vi "Periodic Tasks.vi"(7 "Chassis X SPD":dbl=0.65, 8 "error in":errorcluster) -> ()   [LabVIEW 2019]
doc: "This VI runs in parallel to other tasks. It can contain as many user-defined periodic loops as you need. These can carry out PID or other sorts of timed response."
uses:
  Robot Global Data.vi
  <vilib>/Rock Robotics/Network Tables/NT Write Number.vi
  <vilib>/Analysis/NI_AALPro.lvlib
  <vilib>/Rock Robotics/Network Tables/NT Write Boolean.vi
  <vilib>/Rock Robotics/WPI/RobotDrive/WPI_RobotDriveArcadeDrive_Standard(NoSaturation).vi
  <vilib>/Rock Robotics/Network Tables/NT Read Number.vi
panel:
  in  "Chassis Y SPD":dbl=0.65
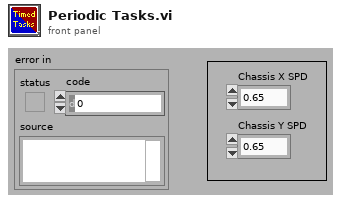
[diagram p1: front panel]
types:
  T1 = typedef "WPI_MotorControlDeviceRef.ctl" = cluster{"DeviceStatus":errorcluster, "Type":T2, "PWM":cluster{"PWM Channel":T3, "DeadBand":T4}, "CAN":cluster{"Device Number":u8, "SetOutput VI Ref":variant, "GetOutput VI Ref":variant, "Enable VI Ref":variant, "Disable VI Ref":variant, "Data":variant}, "Invert":bool, "DIO PWM":cluster{"PWM \"Enable\" Channel":T3, "DIOChannel":T5, "PWM Rate":dbl}}
  T2 = typedef "WPI_MotorControlType.ctl" = enum16{"PWM", "CAN", "DIO PWM"}
  T3 = typedef "FPGA_DIOPWMChannel.ctl" = enum8{"PWM 0", "PWM 1", "PWM 2", "PWM 3", "PWM 4", "PWM 5", "PWM 6", "PWM 7", "PWM 8", "PWM 9", "PWM MXP 0", "PWM MXP 1", "PWM MXP 2", "PWM MXP 3", "PWM MXP 4", "PWM MXP 5", "PWM MXP 6", "PWM MXP 7", "PWM MXP 8", "PWM MXP 9", "Invalid"}
  T4 = typedef "WPI_PWMDeadband.ctl" = cluster{"Name":string, "maxPositivePwm":i32, "minPositivePwm":i32, "centerPwm":i32, "maxNegativePwm":i32, "minNegativePwm":i32, "angularRange":u16}
  T5 = typedef "FPGA_DIOChannel.ctl" = enum8{"DIO 0", "DIO 1", "DIO 2", "DIO 3", "DIO 4", "DIO 5", "DIO 6", "DIO 7", "DIO 8", "DIO 9", "DIO MXP 0", "DIO MXP 1", "DIO MXP 2", "DIO MXP 3", "DIO MXP 4", "DIO MXP 5", "DIO MXP 6", "DIO MXP 7", "DIO MXP 8", "DIO MXP 9", "DIO MXP 10", "DIO MXP 11", "DIO MXP 12", "DIO MXP 13", "DIO MXP 14", "DIO MXP 15", "SPI Port CS1", "SPI Port CS2", "SPI Port CS3", "SPI Port MISO", "SPI Port MOSI", "Invalid"}
  T6 = typedef "WPI_JoystickDevRef.ctl" = cluster{"Device":T7}
  T7 = typedef "WPI_JoystickDeviceEnum.ctl" = enum16{"USB 0", "USB 1", "USB 2", "USB 3", "USB 4", "USB 5"}
  T8 = typedef "WPI_RobotDriveDevRef.ctl" = cluster{"DevStatus":errorcluster, "Motors[]":T1[], "Square Inputs":bool, "Max Output":dbl}
  T9 = cluster{"JoystickDevRef":T6, "RobotDriveDevRef":T8}
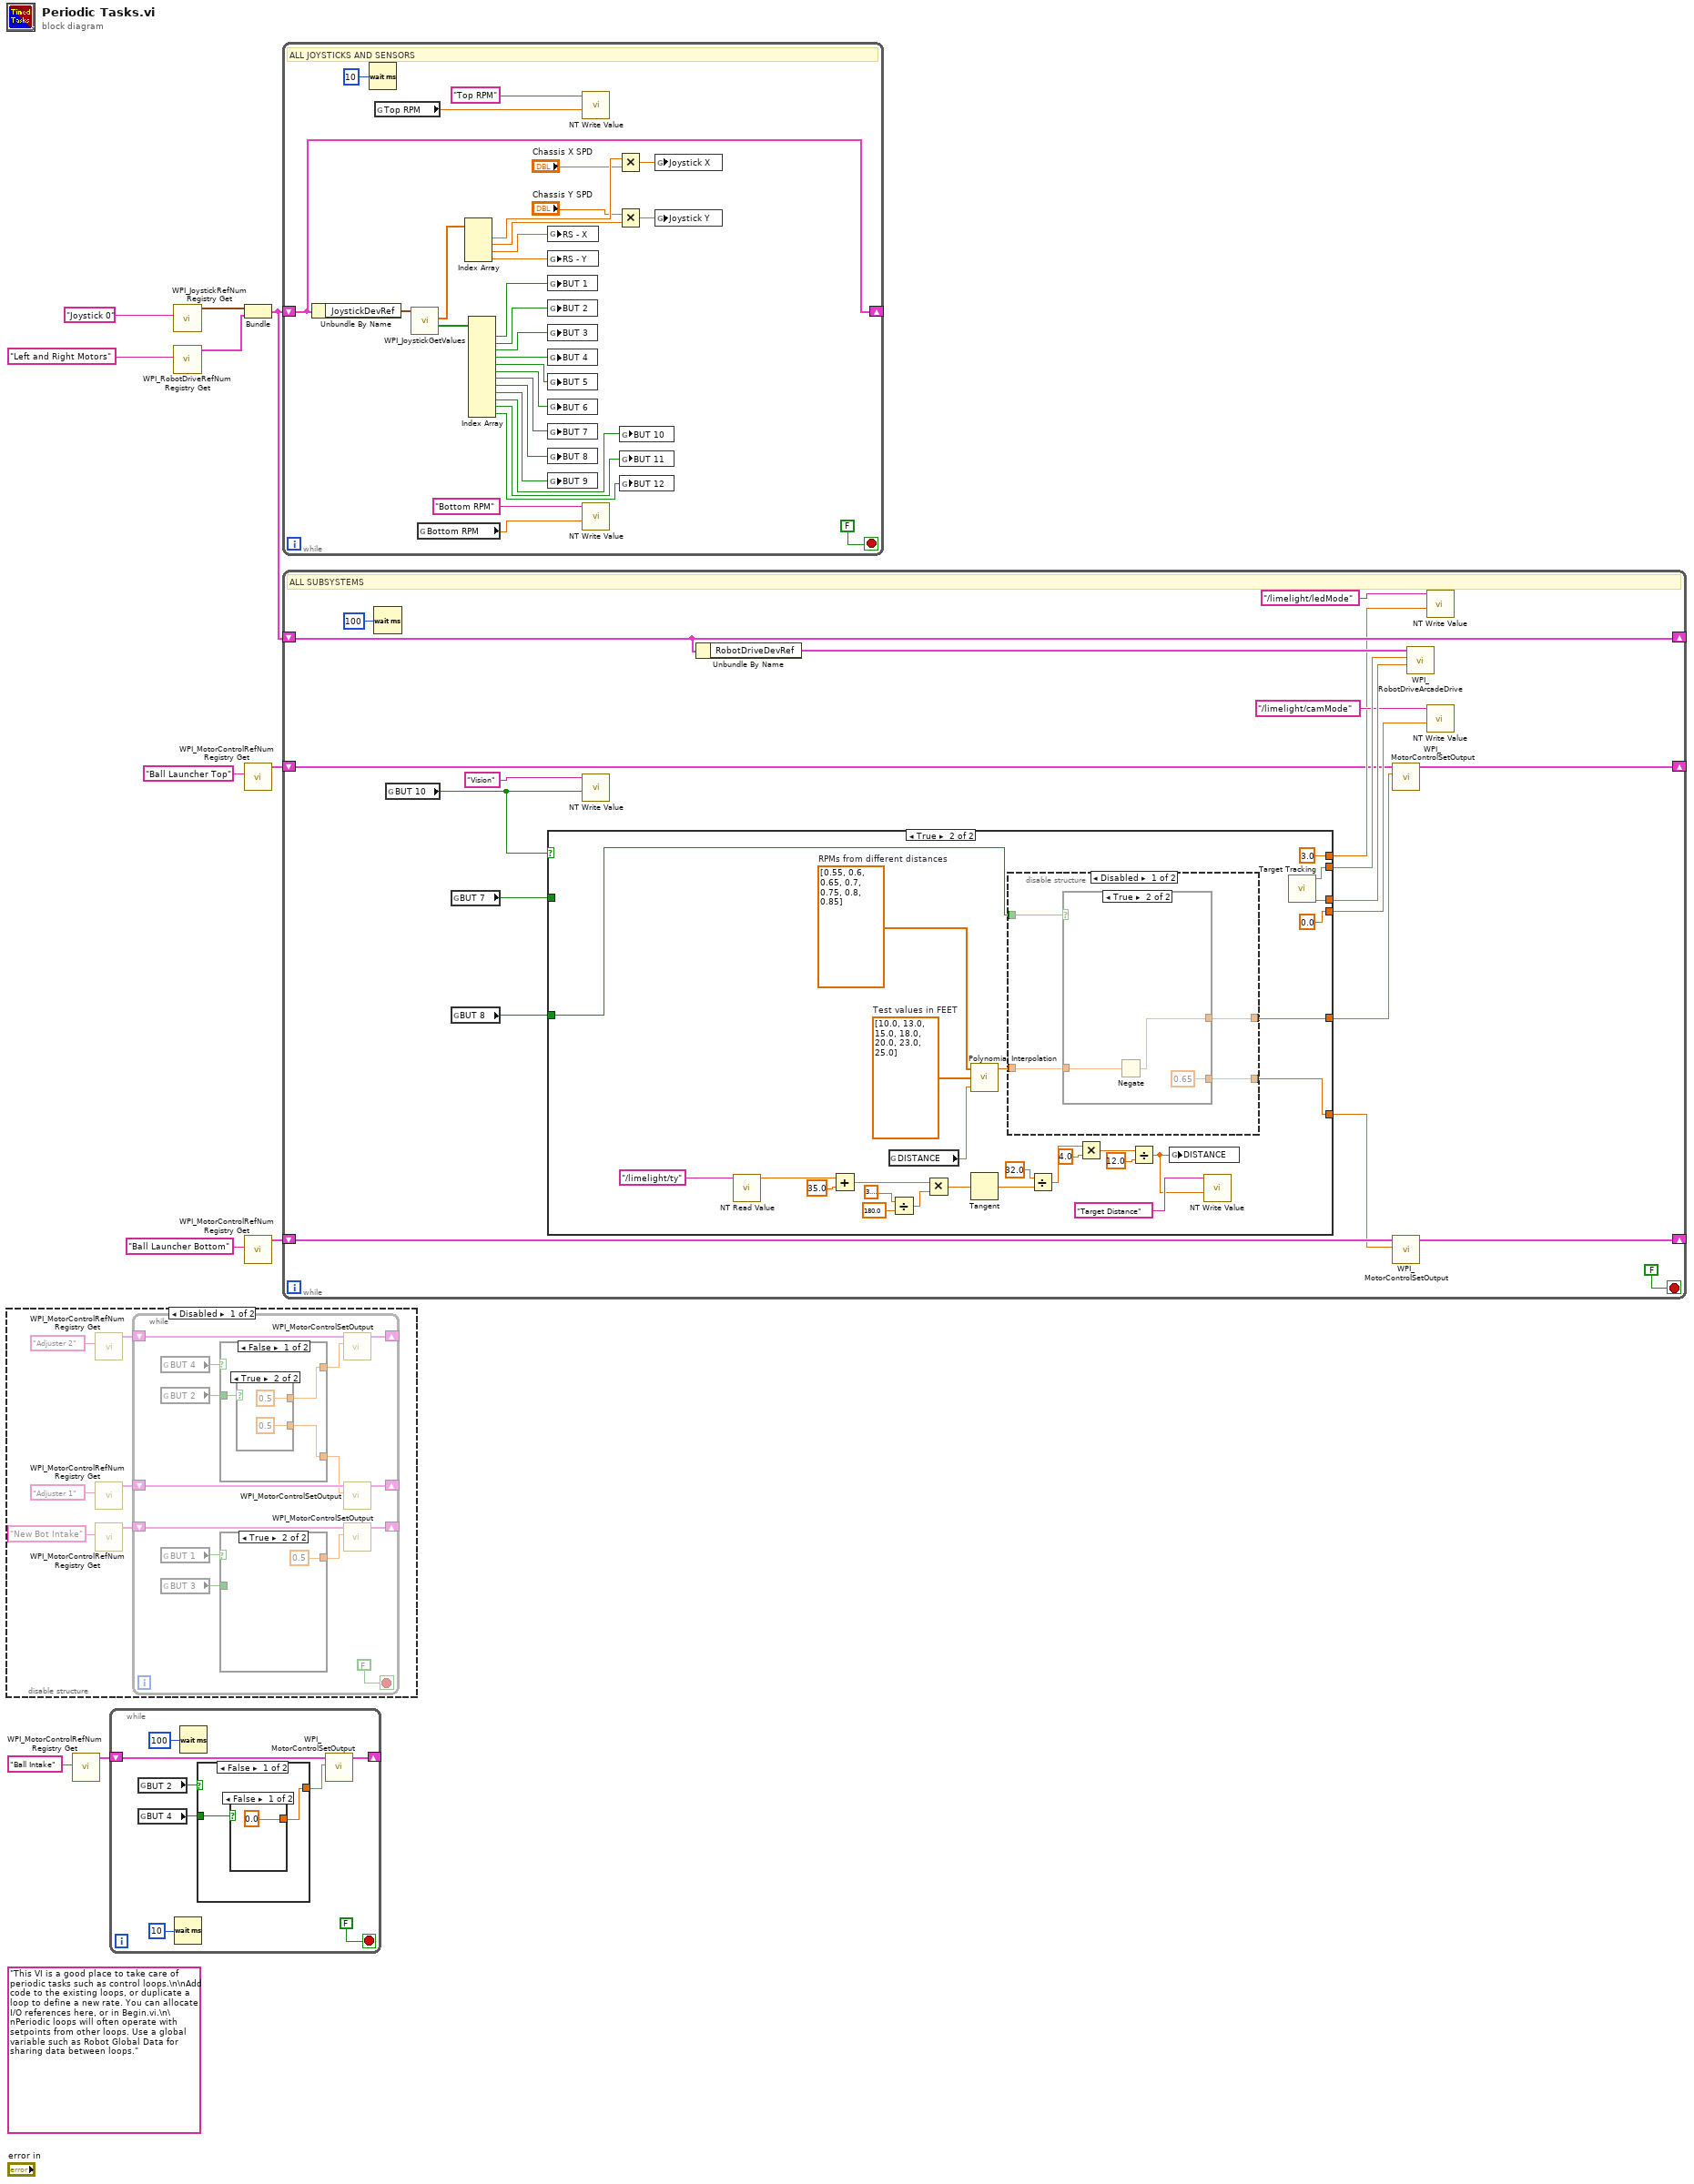
[diagram p0: block diagram]
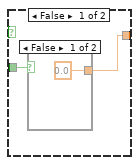
[diagram p2: hidden frame]
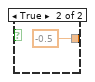
[diagram p3: hidden frame]
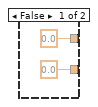
[diagram p4: hidden frame]
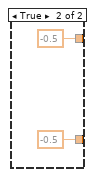
[diagram p5: hidden frame]
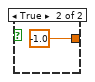
[diagram p7: hidden frame]
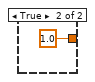
[diagram p8: hidden frame]
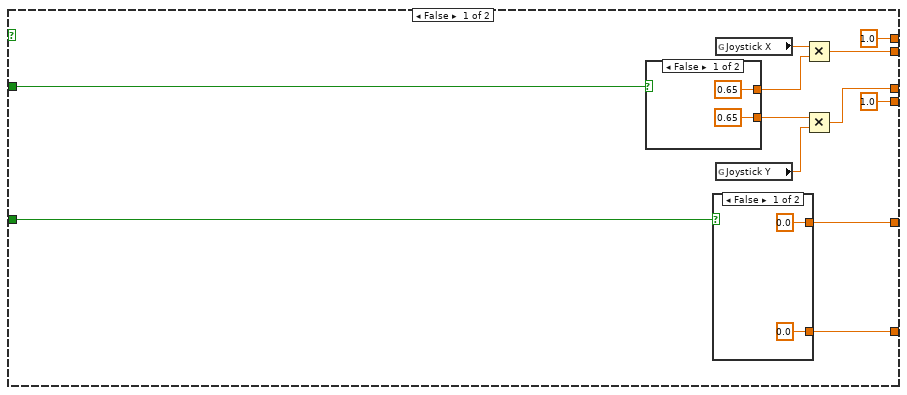
[diagram p9: hidden frame]
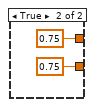
[diagram p10: hidden frame]
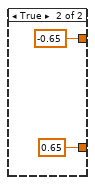
[diagram p11: hidden frame]
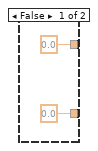
[diagram p12: hidden frame]
diagram:
  (unwired) "This VI is a good place to take care of periodic tasks such as control loops.\n\nAdd code to the existing loops, or duplicate a loop to define a new rate. You can allocate I/O references here, or in Begin.vi.\n\nPeriodic loops will often operate with setpoints from other loops. Use a global variable such as Robot Global Data for sharing data between loops."
  n1 = disable-structure shown="Disabled" {
    frame Disabled {
      n2 = call <vilib>:"WPI_MotorControlRefNum Registry Get.vi"("refnum name"="Adjuster 2") -> ("MotorControlDevRef"=w17:T1)  [unwired: 9 in, 1 out]
      n3 = call <vilib>:"WPI_MotorControlRefNum Registry Get.vi"("refnum name"="Adjuster 1") -> ("MotorControlDevRef"=w14:T1)  [unwired: 9 in, 1 out]
      n4 = call <vilib>:"WPI_MotorControlRefNum Registry Get.vi"("refnum name"="New Bot Intake") -> ("MotorControlDevRef"=w13:T1)  [unwired: 9 in, 1 out]
      n5 = while {
        shift-right: [w30] -> _
        shift-left: w17 -> [w29]
        shift-right: [w28] -> _
        shift-left: w14 -> [w27]
        shift-right: [w21] -> _
        shift-left: w13 -> [w22]
        stop <- FALSE stop-if-true
        n6 = global read "Robot Global Data.vi" "BUT 4"() -> (w26:bool)
        n7 = global read "Robot Global Data.vi" "BUT 2"() -> (w25:bool)
        n8 = global read "Robot Global Data.vi" "BUT 1"() -> (w20:bool)
        n9 = global read "Robot Global Data.vi" "BUT 3"() -> (w18:bool)
        n10 = case shown="False" w26 {
          tunnel: [w39 -0.5 ("Output")] -> w24
          tunnel: w25 -> [w38 _]
          tunnel: [w37 -0.5 ("Output")] -> w23
          frame False {
            n11 = case shown="True" w38 {
              tunnel: [0.0 ("Output") 0.5 ("Output")] -> w39
              tunnel: [0.0 ("Output") 0.5 ("Output")] -> w37
              frame False {
              }
              frame True {
              }
            }
          }
          frame True {
          }
        }
        n12 = case shown="True" w20 {
          tunnel: [w33 0.5 ("Output")] -> w19
          tunnel: w18 -> [w32 _]
          frame False {
            n13 = case shown="False" w32 {
              tunnel: [0.0 ("Output") -0.5 ("Output")] -> w33
              frame False {
              }
              frame True {
              }
            }
          }
          frame True {
          }
        }
        n14 = call <vilib>:"WPI_MotorControlSetOutput.vi"("Output"=w24, "MotorControlDevRef"=w29) -> ("MotorControlDevRef"=w30:T1)  [unwired: 7 in, 2 out]
        n15 = call <vilib>:"WPI_MotorControlSetOutput.vi"("Output"=w23, "MotorControlDevRef"=w27) -> ("MotorControlDevRef"=w28:T1)  [unwired: 7 in, 2 out]
        n16 = call <vilib>:"WPI_MotorControlSetOutput.vi"("Output"=w19, "MotorControlDevRef"=w22) -> ("MotorControlDevRef"=w21:T1)  [unwired: 7 in, 2 out]
      }
    }
    frame Enabled {
    }
  }
  n17 = call <vilib>:"WPI_MotorControlRefNum Registry Get.vi"("refnum name"="Ball Intake") -> ("MotorControlDevRef"=w6:T1)  [unwired: 9 in, 1 out]
  n18 = while {
    shift-right: [w50] -> _
    shift-left: w6 -> [w49]
    stop <- FALSE stop-if-true
    n19 = global read "Robot Global Data.vi" "BUT 2"() -> (w52:bool)
    n20 = global read "Robot Global Data.vi" "BUT 4"() -> (w53:bool)
    n21 = Wait (ms)(milliseconds to wait=u32 10) -> ()  [unwired: 1 out]
    n22 = Wait (ms)(milliseconds to wait=u32 100) -> ()  [unwired: 1 out]
    n23 = case shown="False" w52 {
      tunnel: [w55 1.0 ("Output")] -> w51
      tunnel: w53 -> [w54 _]
      frame False {
        n24 = case shown="False" w54 {
          tunnel: [0.0 ("Output") -1.0 ("Output")] -> w55
          frame False {
          }
          frame True {
          }
        }
      }
      frame True {
      }
    }
    n25 = call <vilib>:"WPI_MotorControlSetOutput.vi"("Output"=w51, "MotorControlDevRef"=w49) -> ("MotorControlDevRef"=w50:T1)  [unwired: 7 in, 2 out]
  }
  n26 = call <vilib>:"WPI_JoystickRefNum Registry Get.vi"("refnum name"="Joystick 0") -> ("JoystickDevRef"=w9:T6)  [unwired: 1 in, 9 out]
  n27 = call <vilib>:"WPI_RobotDriveRefNum Registry Get.vi"("refnum name"="Left and Right Motors") -> ("RobotDriveDevRef"=w8:T8)  [unwired: 1 in, 9 out]
  n28 = Bundle("JoystickDevRef"=w9, "RobotDriveDevRef"=w8) -> (w7:T9)  [unwired: 1 out]
  n29 = call <vilib>:"WPI_MotorControlRefNum Registry Get.vi"("refnum name"="Ball Launcher Top") -> ("MotorControlDevRef"=w4:T1)  [unwired: 9 in, 1 out]
  n30 = call <vilib>:"WPI_MotorControlRefNum Registry Get.vi"("refnum name"="Ball Launcher Bottom") -> ("MotorControlDevRef"=w1:T1)  [unwired: 9 in, 1 out]
  n31 = while {
    shift-right: [w73] -> _
    shift-left: w7 -> [w73]
    stop <- FALSE stop-if-true
    # "ALL JOYSTICKS AND SENSORS"
    n32 = Unbundle By Name(w73) -> ("JoystickDevRef"=w87:T6)
    n33 = Wait (ms)(milliseconds to wait=u32 10) -> ()  [unwired: 1 out]
    n34 = global read "Robot Global Data.vi" "Top RPM"() -> (w59:dbl)
    n35 = call <vilib>:"WPI_JoystickGetValues.vi"("JoystickDevRef"=w87) -> ("Buttons"=w86:bool[], "Axes"=w72:dbl[])  [unwired: 6 in, 3 out]
    n36 = global read "Robot Global Data.vi" "Bottom RPM"() -> (w61:dbl)
    n37 = Index Array(array=w72) -> (element #1=w69:dbl, element #2=w68:dbl, element #3=w65:dbl, element #4=w64:dbl)  [unwired: 4 in]
    n38 = Index Array(array=w86) -> (element #1=w85:bool, element #2=w84:bool, element #3=w83:bool, element #4=w82:bool, element #5=w81:bool, element #6=w80:bool, element #7=w79:bool, element #8=w78:bool, element #9=w77:bool, element #10=w76:bool, element #11=w75:bool, element #12=w74:bool)  [unwired: 12 in]
    n39 = global write "Robot Global Data.vi" "RS - X"(w65) -> ()
    n40 = global write "Robot Global Data.vi" "RS - Y"(w64) -> ()
    n41 = global write "Robot Global Data.vi" "BUT 1"(w85) -> ()
    n42 = global write "Robot Global Data.vi" "BUT 2"(w84) -> ()
    n43 = global write "Robot Global Data.vi" "BUT 3"(w83) -> ()
    n44 = global write "Robot Global Data.vi" "BUT 4"(w82) -> ()
    n45 = global write "Robot Global Data.vi" "BUT 5"(w81) -> ()
    n46 = global write "Robot Global Data.vi" "BUT 6"(w80) -> ()
    n47 = global write "Robot Global Data.vi" "BUT 7"(w79) -> ()
    n48 = global write "Robot Global Data.vi" "BUT 8"(w78) -> ()
    n49 = global write "Robot Global Data.vi" "BUT 9"(w77) -> ()
    n50 = call-poly <vilib>:"NT Write Value.vi"("Numeric"=w59, "Name"="Top RPM") -> ()  [unwired: 9 in, 1 out]
    n51 = call-poly <vilib>:"NT Write Value.vi"("Numeric"=w61, "Name"="Bottom RPM") -> ()  [unwired: 9 in, 1 out]
    n52 = Multiply(x=w69, y="Chassis X SPD") -> (x*y=w71:dbl)
    n53 = Multiply(x="Chassis Y SPD", y=w68) -> (x*y=w70:dbl)
    n54 = global write "Robot Global Data.vi" "BUT 10"(w76) -> ()
    n55 = global write "Robot Global Data.vi" "BUT 11"(w75) -> ()
    n56 = global write "Robot Global Data.vi" "BUT 12"(w74) -> ()
    n57 = global write "Robot Global Data.vi" "Joystick X"(w71) -> ()
    n58 = global write "Robot Global Data.vi" "Joystick Y"(w70) -> ()
  }
  n59 = while {
    shift-right: [w107] -> _
    shift-left: w7 -> [w107]
    shift-right: [w89] -> _
    shift-left: w4 -> [w97]
    shift-right: [w90] -> _
    shift-left: w1 -> [w96]
    stop <- FALSE stop-if-true
    # "ALL SUBSYSTEMS"
    n60 = Wait (ms)(milliseconds to wait=u32 100) -> ()  [unwired: 1 out]
    n61 = global read "Robot Global Data.vi" "BUT 10"() -> (w98:bool)
    n62 = global read "Robot Global Data.vi" "BUT 7"() -> (w92:bool)
    n63 = global read "Robot Global Data.vi" "BUT 8"() -> (w93:bool)
    n64 = case shown="True" w98 {
      tunnel: [w115 w130] -> w105
      tunnel: [w114 w129] -> w104
      tunnel: [1.0 ("Numeric") 0.0 ("Numeric")] -> w101
      tunnel: [1.0 ("Numeric") 3.0 ("Numeric")] -> w100
      tunnel: [w118 w134] -> w95
      tunnel: [w117 w132] -> w94
      tunnel: w93 -> [w116 w131]
      tunnel: w92 -> [w109 _]
      frame False {
        n65 = case shown="False" w109 {
          tunnel: [0.65 ("x") 0.75 ("x")] -> w111
          tunnel: [0.65 ("y") 0.75 ("y")] -> w110
          frame False {
          }
          frame True {
          }
        }
        n66 = case shown="False" w116 {
          tunnel: [0.0 ("Output") -0.65 ("Output")] -> w118
          tunnel: [0.0 ("Output") 0.65 ("Output")] -> w117
          frame False {
          }
          frame True {
          }
        }
        n67 = global read "Robot Global Data.vi" "Joystick X"() -> (w112:dbl)
        n68 = global read "Robot Global Data.vi" "Joystick Y"() -> (w113:dbl)
        n69 = Multiply(x=w112, y=w110) -> (x*y=w115:dbl)
        n70 = Multiply(x=w111, y=w113) -> (x*y=w114:dbl)
      }
      frame True {
        w137 = dbl[] [10.0, 13.0, 15.0, 18.0, 20.0, 23.0, 25.0]  # Test values in FEET
        w138 = dbl[] [0.55, 0.6, 0.65, 0.7, 0.75, 0.8, 0.85]  # RPMs from different distances
        n71 = call-poly <vilib>:"NT Read Value.vi"("Name"="/limelight/ty") -> ("Numeric"=w148:dbl)  [unwired: 9 in, 1 out]
        n72 = Add(x=w148, y=35.0) -> (x+y=w146:dbl)
        n73 = global read "Robot Global Data.vi" "DISTANCE"() -> (w135:dbl)
        n74 = Divide(x=3.141592653589793, y=180.0) -> (x/y=w149:dbl)
        n75 = Multiply(x=w146, y=w149) -> (x*y=w145:dbl)
        n76 = call <vilib>:"Polynomial Interpolation.vi"("x value"=w135, "X"=w137, "Y"=w138) -> ("interpolation value"=w133:dbl)  [unwired: 2 out]
        n77 = Tangent(1:w145) -> (0:w155:dbl)
        n78 = disable-structure shown="Disabled" {
          disable-tunnel: [w159 _] -> w134
          disable-tunnel: w133 -> [w158 _]
          disable-tunnel: [w157 _] -> w132
          disable-tunnel: w131 -> [w156 _]
          frame Disabled {
            n79 = case shown="True" w156 {
              tunnel: [0.0 w164] -> w159
              tunnel: w158 -> [_ w163]
              tunnel: [0.0 ("Output") 0.65 ("Output")] -> w157
              frame False {
              }
              frame True {
                n80 = Negate(x=w163) -> (-x=w164:dbl)
              }
            }
          }
          frame Enabled {
          }
        }
        n81 = Divide(x=32.0, y=w155) -> (x/y=w144:dbl)
        n82 = Multiply(x=w144, y=4.0) -> (x*y=w142:dbl)
        n83 = Divide(x=w142, y=12.0) -> (x/y=w136:dbl)
        n84 = global write "Robot Global Data.vi" "DISTANCE"(w136) -> ()
        n85 = call-poly <vilib>:"NT Write Value.vi"("Numeric"=w136, "Name"="Target Distance") -> ()  [unwired: 9 in, 1 out]
        n86 = call "Target Tracking.vi"() -> ("Joystick Y"=w129:dbl, "Joystick X"=w130:dbl)  [unwired: 10 in]
      }
    }
    n87 = call-poly <vilib>:"NT Write Value.vi"("Boolean"=w98, "Name"="Vision") -> ()  [unwired: 9 in, 1 out]
    n88 = Unbundle By Name(w107) -> ("RobotDriveDevRef"=w106:T8)
    n89 = call <vilib>:"WPI_MotorControlSetOutput.vi"("Output"=w95, "MotorControlDevRef"=w97) -> ("MotorControlDevRef"=w89:T1)  [unwired: 7 in, 2 out]
    n90 = call <vilib>:"WPI_MotorControlSetOutput.vi"("Output"=w94, "MotorControlDevRef"=w96) -> ("MotorControlDevRef"=w90:T1)  [unwired: 7 in, 2 out]
    n91 = call-poly <vilib>:"WPI_RobotDriveArcadeDrive.vi"("Y axis value"=w104, "X axis value"=w105, "RobotDriveDevRef"=w106) -> ()  [unwired: 6 in, 3 out]
    n92 = call-poly <vilib>:"NT Write Value.vi"("Numeric"=w100, "Name"="/limelight/ledMode") -> ()  [unwired: 9 in, 1 out]
    n93 = call-poly <vilib>:"NT Write Value.vi"("Numeric"=w101, "Name"="/limelight/camMode") -> ()  [unwired: 9 in, 1 out]
  }
